vi "Set Strain.vi"(6 "Channel":i32=1 min=1 max=2, 8 "error in (no error)":errorcluster, 9 "Slew (V/s)":dbl, 10 "Strain (V)":dbl, 11 "Inst.RP100 in":refnum<class "Inst.RP100.lvclass">) -> (0 "error out":errorcluster, 3 "Inst.RP100 out":refnum<class "Inst.RP100.lvclass">)   [LabVIEW 2019, in "Inst.RP100.lvlib" / "Inst.RP100.lvclass"]
doc: "Set the output <b>Strain</b> with <b>Slew</b> such that Channel 1 = -Channel 2. \n\n<b>Output Channel</b> is not used."
uses:
  Inst.RP100.lvclass
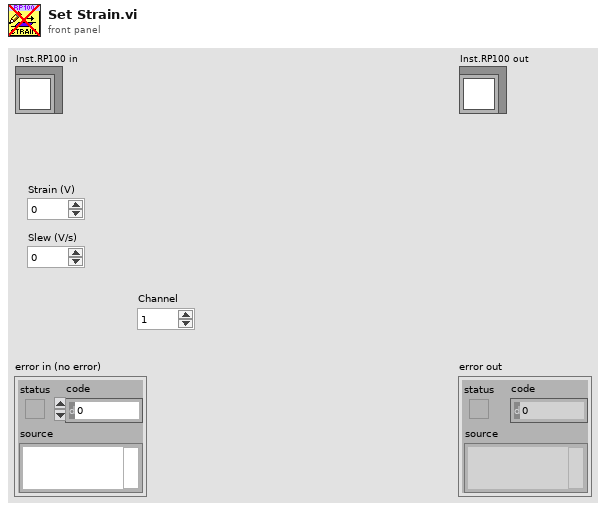
[diagram p1: front panel]
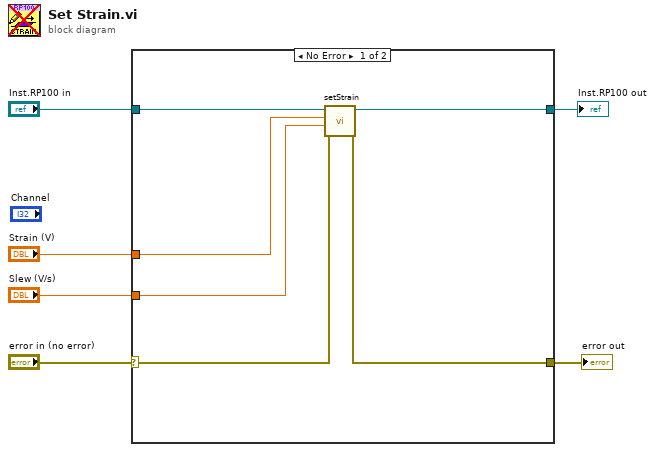
[diagram p0: block diagram]
diagram:
  n1 = case shown="No Error" "error in (no error)" {
    selector: "error in (no error)" -> [w9 w14]
    tunnel: [w8 w14] -> w5
    tunnel: "Strain (V)" -> [w11 _]
    tunnel: "Inst.RP100 in" -> [w12 w13]
    tunnel: [w7 w13] -> w2
    tunnel: "Slew (V/s)" -> [w10 _]
    frame No Error {
      n2 = call-dynamic "setStrain.vi"("error in (no error)"=w9, "Slew (V/s)"=w10, "Strain (V)"=w11, "Inst.RP100 in"=w12) -> ("error out"=w8:errorcluster, "Inst.RP100 out"=w7:refnum<class "Inst.RP100.lvclass">)  [unwired: 6 in]
    }
    frame Error {
    }
  }
  "error out" <- w5
  "Inst.RP100 out" <- w2
